vi "FGV_MacroExecStep.vi"() -> ()   [LabVIEW 2012]
panel:
  out "Error Out":errorcluster
  in  "Error In":errorcluster
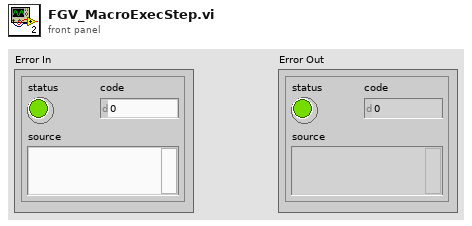
[diagram p1: front panel]
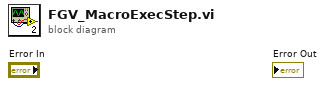
[diagram p0: block diagram]
diagram:
